vi "fgt set purge.vi"(8 "error in (no error)":errorcluster, 10 "purge":bool, 11 "controllerIndex":u16) -> (0 "error out":errorcluster)   [LabVIEW 2016, in "fgt_SDK.lvlib"]
doc: "Activate/deactivate purge function.\nThis feature is only available on MFCS devices equipped with special valve."
uses:
  fgt_SDK.lvlib
  dlls/fgt_SDK_32.dll
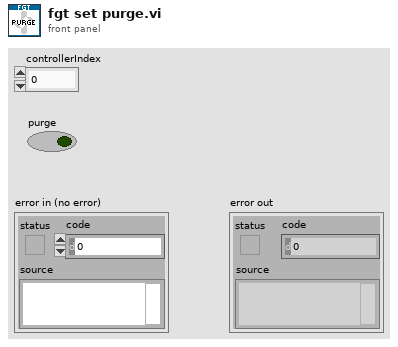
[diagram p1: front panel]
types:
  T1 = typedef "fgt_SDK.lvlib/fgt_STATUS_INFO.ctl" = cluster{"InstrType":T2, "instrSN":u16, "errorCode":u8, "infoCode":u8, "detail":string}
  T2 = typedef "fgt_SDK.lvlib/fgt_INSTRUMENT_TYPE.ctl" = enum32{"None", "MFCS", "MFCS_EZ", "FRP", "LineUP"}
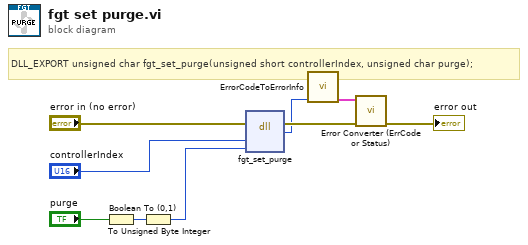
[diagram p0: block diagram]
diagram:
  # "DLL_EXPORT unsigned char fgt_set_purge(unsigned short controllerIndex, unsigned char purge);"
  n1 = Boolean To (0,1)(Boolean="purge") -> (0, 1=w5:i16)
  n2 = To Unsigned Byte Integer(number=w5) -> (unsigned 8bit integer=w3:u8)
  n3 = dll-call lib="PTH2Zabs D\nMes DocumentsDéveloppementFluigentSDKsfgt-sdk-labviewdllsfgt_SDK_*.*" fn="fgt_set_purge"(error in="error in (no error)", "controllerIndex"="controllerIndex", "purge"=w3) -> (error out=w7:errorcluster, "return type"=w2:u8)  [unwired: 4 in, 1 out]
  n4 = call "ErrorCodeToErrorInfo.vi"("return type"=w2) -> ("StatusInfo"=w1:T1)  [unwired: 10 in]
  n5 = call "Error Converter (ErrCode or Status).vi"("error in (no error)"=w7, "StatusInfo"=w1) -> ("error out"=→"error out":errorcluster)  [unwired: 9 in]
